vi "Render.vi"(7 "Renderer":refnum<class "Renderer.lvclass">, 8 "error in (no error)":errorcluster, 10 "Camera":refnum<class "Camera.lvclass">, 11 "Chmmr in":refnum<class "Chmmr.lvclass">) -> (0 "error out":errorcluster)   [LabVIEW 2021, in "Chmmr.lvclass"]
uses:
  Chmmr.lvclass
  Camera/Camera.lvclass
  Renderer/Renderer.lvclass
  Ship/Ship.lvclass
  LabSDL2/Source/Libraries/LibSDL2 Wrapper/LibSDL2.lvlib
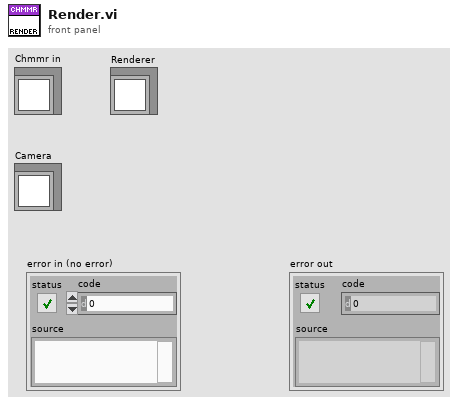
[diagram p1: front panel]
types:
  T1 = typedef "LibSDL2.lvlib/Rectangle.ctl" = cluster{"x":i32, "y":i32, "Width":i32, "Height":i32}
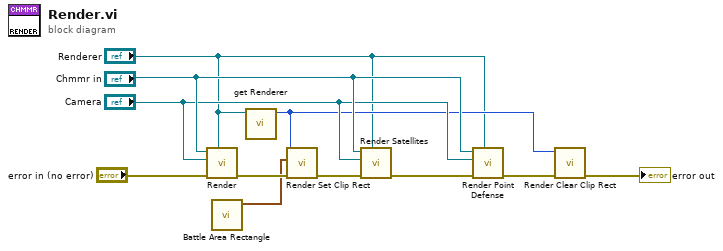
[diagram p0: block diagram]
diagram:
  n1 = call-parent "Render.vi"("Renderer"="Renderer", "error in (no error)"="error in (no error)", "Camera"="Camera", "Ship in"="Chmmr in") -> ("error out"=w7:errorcluster)  [unwired: 7 in]
  n2 = call "Battle Area Rectangle.vi"() -> ("Viewport"=w1:T1)  [unwired: 11 in]
  n3 = call-dynamic "get Renderer.vi"("Renderer in"="Renderer") -> ("Renderer"=w3:u32)  [unwired: 10 in]
  n4 = call "Render Set Clip Rect.vi"("error in"=w7, "Rectangle"=w1, "Renderer Pointer"=w3) -> ("error out"=w4:errorcluster)  [unwired: 7 in, 1 out]
  n5 = call "Render Satellites.vi"("Renderer"="Renderer", "error in (no error)"=w4, "Camera"="Camera", "Chmmr in"="Chmmr in") -> ("error out"=w9:errorcluster)  [unwired: 7 in]
  n6 = call "Render Point Defense.vi"("Renderer"="Renderer", "error in (no error)"=w9, "Camera"="Camera", "Chmmr in"="Chmmr in") -> ("error out"=w6:errorcluster)  [unwired: 7 in]
  n7 = call "Render Clear Clip Rect.vi"("error in"=w6, "Renderer Pointer"=w3) -> ("error out"=→"error out":errorcluster)  [unwired: 8 in, 1 out]
